vi "SetOccurance.vi"(1 "Occurrence Refnum":refnum<k4>, 2 "String Input Refnum":refnum<vi>, 3 "Input String":string, 4 "Number O fTimes To Loop":u32) -> ()   [LabVIEW 2010]
panel:
  out "Counter":u32
  out "String 2":string
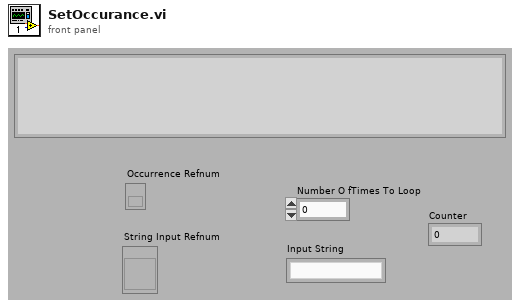
[diagram p1: front panel]
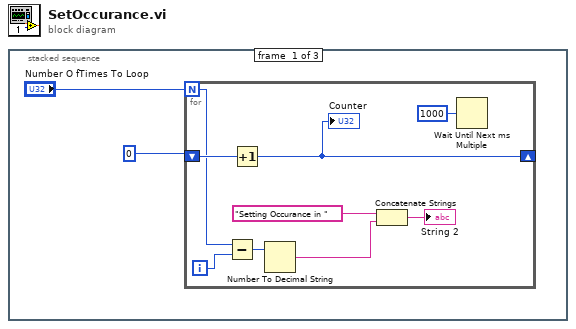
[diagram p0: block diagram]
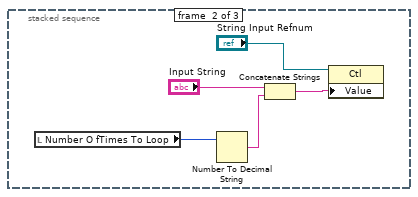
[diagram p2: hidden frame]
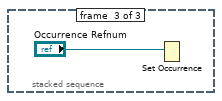
[diagram p3: hidden frame]
diagram:
  n1 = stacked-sequence {
    frame #0 {
      n2 = for {
        N: "Number O fTimes To Loop" -> [w3]
        shift-right: [w6] -> _
        shift-left: u32 0 -> [w7]
        i -> [w4]
        n3 = Subtract(x=w3, y=w4) -> (x-y=w5:i32)
        n4 = Increment(x=w7) -> (x+1=w6:u32)
        "Counter" <- w6
        n5 = Number To Decimal String(number=w5) -> (decimal integer string=w8:string)  [unwired: 1 out]
        n6 = Concatenate Strings("Setting Occurance in ", w8) -> (→"String 2":string)
        n7 = Wait Until Next ms Multiple(millisecond multiple=u32 1000) -> ()  [unwired: 1 out]
      }
    }
    frame #1 {
      n8 = local read "Number O fTimes To Loop"() -> (w13:u32)
      n9 = Number To Decimal String(number=w13) -> (decimal integer string=w15:string)  [unwired: 1 out]
      n10 = Concatenate Strings("Input String", w15) -> (w12:string)
      n11 = property class="Ctl"(reference="String Input Refnum", "Value"=w12) -> ()  [unwired: 1 in, 2 out]
    }
    frame #2 {
      n12 = Set Occurrence("Occurrence Refnum") -> ()
    }
  }
